vi "Get Session Property (Core).vi"(0 "SLSC Remote in":refnum<class "SLSC Remote.lvclass">, 11 "error in (no error)":errorcluster) -> (4 "SLSC Remote out":refnum<class "SLSC Remote.lvclass">, 15 "error out":errorcluster)   [LabVIEW 2015, in "SLSC Remote.lvclass"]
uses:
  SLSC Remote.lvclass
  SLSC Interface Class/SLSC Interface.lvclass
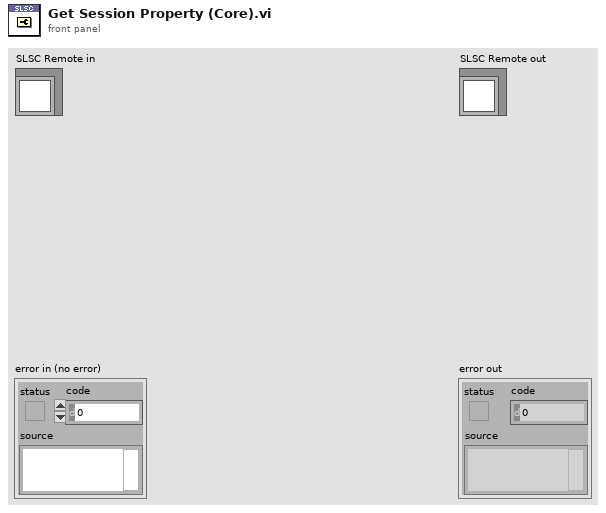
[diagram p1: front panel]
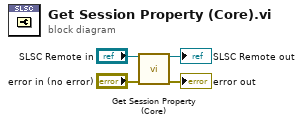
[diagram p0: block diagram]
diagram:
  n1 = call-parent "Get Session Property (Core).vi"("SLSC Interface in"="SLSC Remote in", "error in (no error)"="error in (no error)") -> ("SLSC Interface out"=→"SLSC Remote out":refnum<class "SLSC Remote.lvclass">, "error out"=→"error out":errorcluster)  [unwired: 12 in]
